vi "Write.vi"() -> ()   [LabVIEW 2023]
uses:
  <vilib>/OPCUA/controls/NodeId.ctl
  <vilib>/OPCUA/controls/Write Status.ctl
  <vilib>/OPCUA/NI OPC UA Client.lvlib
  <vilib>/OPCUA/client/Multiple Write Double.vi
panel:
  out "Temperature from DAQ":dbl
  in  "Stop Button":bool
  in  "Item Path":string="ns=2;s=Tag1"
  in  "Server Endpoint URL":string="opc.tcp://beist:62640/IntegrationObjects/ServerSimulator"
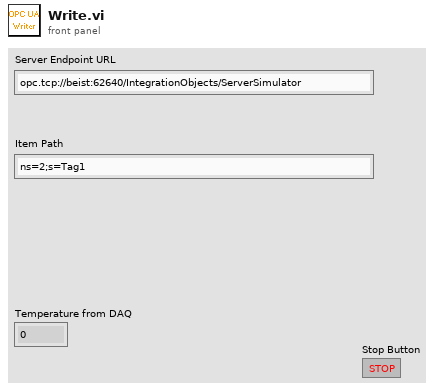
[diagram p1: front panel]
types:
  T1 = cluster{"message mode":enum16{"None", "Sign", "Sign and Encrypt"}, "security":enum16{"Basic256", "Basic128Rsa15"}}
  T2 = typedef "OPC UA Client Refnum.ctl" = refnum<k21>
  T3 = typedef "NodeId.ctl" = string
  T4 = typedef "Write Status.ctl" = u32
  T5 = cluster{"node ID":T3, "value":dbl, "timestamp (current time)":timestamp, "node status":T4}
  T6 = cluster{"node ID":T3, "value":dbl, "timestamp (current time)":timestamp, "node status":T4}[]
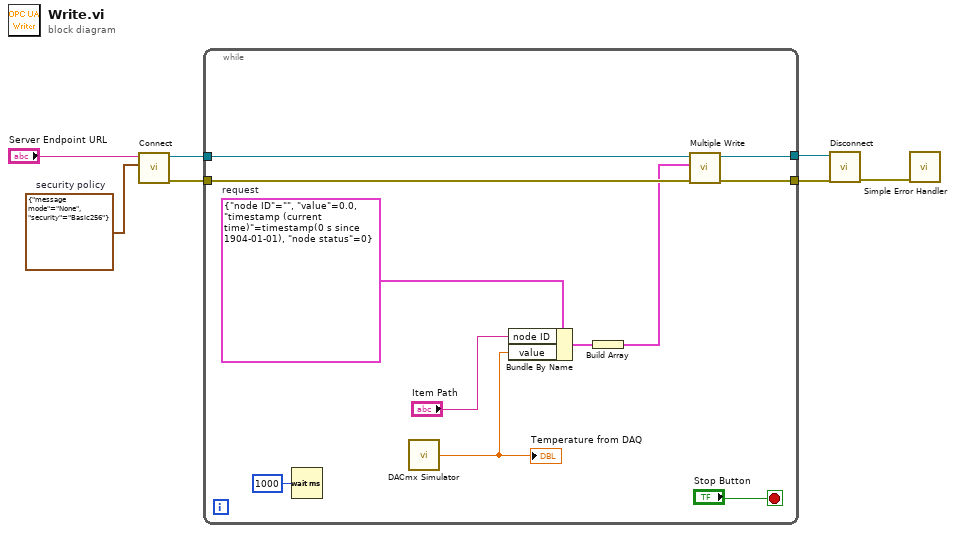
[diagram p0: block diagram]
diagram:
  w7 = T1 {"message mode"=enum."None", "security"=enum."Basic256"}  # security policy
  n1 = call <vilib>:"Connect.vi"("security policy"=w7, "server endpoint URL"="Server Endpoint URL") -> ("error out"=w4:errorcluster, "OPC UA client refnum out"=w6:T2)  [unwired: 7 in, 1 out]
  n2 = while {
    tunnel: w6 -> [w16]
    tunnel: [w15] -> w5
    tunnel: w4 -> [w14]
    tunnel: [w13] -> w3
    stop <- "Stop Button" stop-if-true
    w10 = T5 {"node ID"="", "value"=0.0, "timestamp (current time)"=timestamp(0 s since 1904-01-01), "node status"=0}  # request
    n3 = Wait (ms)(milliseconds to wait=u32 1000) -> ()  [unwired: 1 out]
    n4 = call "DACmx Simulator.vi"() -> ("Analog Input"=w8:dbl)  [unwired: 1 in]
    "Temperature from DAQ" <- w8
    n5 = Bundle By Name "Bundle By Name"(cluster=w10, "node ID"="Item Path", "value"=w8) -> (w11:T5)
    n6 = Build Array "Build Array"(w11) -> (w9:T6)
    n7 = call-poly <vilib>:"Multiple Write.vi"("error in (no error)"=w14, "requests"=w9, "OPC UA client refnum in"=w16) -> ("error out"=w13:errorcluster, "OPC UA client refnum out"=w15:T2)  [unwired: 5 in, 2 out]
  }
  n8 = call <vilib>:"Disconnect.vi"("error in (no error)"=w3, "OPC UA client refnum in"=w5) -> ("error out"=w2:errorcluster)  [unwired: 9 in]
  n9 = call <vilib>:"Simple Error Handler.vi"("error in (no error)"=w2) -> ()  [unwired: 4 in, 5 out]
